vi "GetDemModeStr.vi"(8 "错误输入（无错误）":errorcluster, 9 "检波模式索引":u8, 10 "字符串分配空间大小":u32, 11 "检波模式描述":string) -> (0 "错误输出":errorcluster)   [LabVIEW 2014]
uses:
  X86Dll/ZXUTConfigMgr.dll
panel:
  out "检波模式描述":string
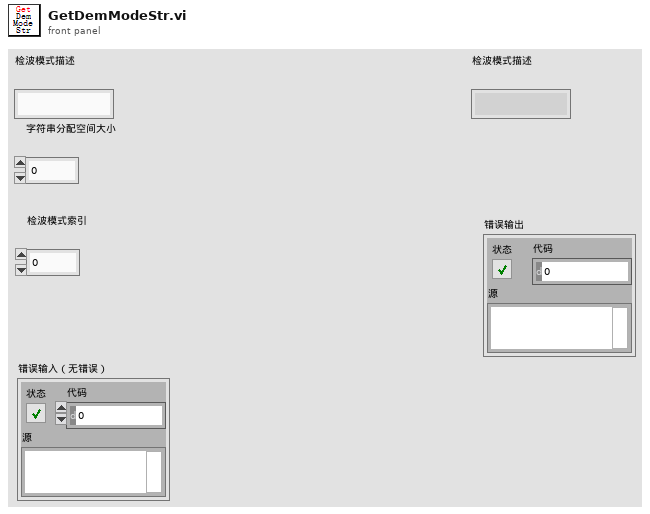
[diagram p1: front panel]
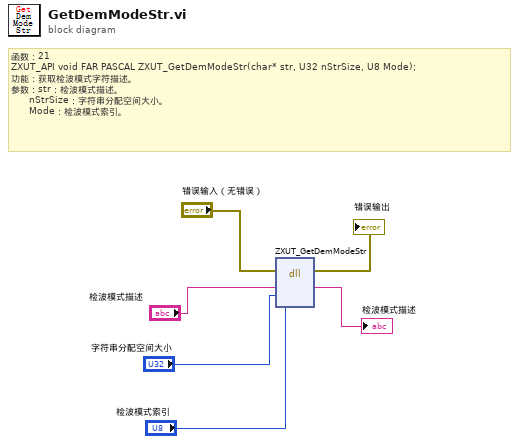
[diagram p0: block diagram]
diagram:
  # "函数：21\nZXUT_API void\tFAR PASCAL ZXUT_GetDemModeStr(char* str, U32 nStrSize, U8 Mode);\n功能：获取检波模式字符描述。\n参数：str：检波模式描述。\n      nStrSize：字符串分配空间大小。\n      Mode：检波模式索引。"
  n1 = dll-call lib="D:/Software/Utrasonic on-line monitoring/X86Dll/ZXUTConfigMgr.dll" fn="ZXUT_GetDemModeStr"(error in="错误输入（无错误）", "str"="检波模式描述", "nStrSize"="字符串分配空间大小", "Mode"="检波模式索引") -> (error out=→"错误输出":errorcluster, "str"=→"检波模式描述":string)  [unwired: 5 in, 1 out]
